vi "T-Periodic Square Gate.vi"(4 "Period T":dbl format="%#_4g", 9 "W":dbl format="%#_4g", 11 "t":dbl format="%#_4g") -> (3 "Square(t)":dbl format="%#_4g")   [LabVIEW 2021, in "Math.lvlib"]
uses:
  Math.lvlib
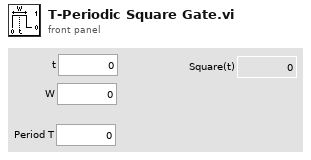
[diagram p1: front panel]
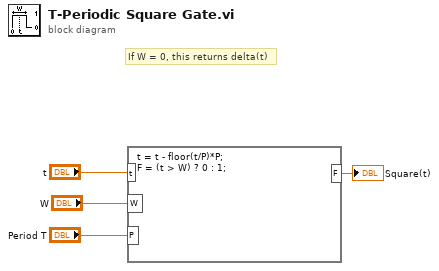
[diagram p0: block diagram]
diagram:
  # "If W = 0, this returns delta(t)"
  n1 = formula code="t = t - floor(t/P)*P;\nF = (t > W) ? 0 : 1;"("t"="t", "W"="W", "P"="Period T") -> ("F"=→"Square(t)":dbl)
